vi "Get COM Descriptor from VISA.vi"(8 "error in (no error)":errorcluster, 10 "Generate error if no COM port found? (False)":bool, 11 "VISA resource name":refnum<visa-resource-name>) -> (0 "error out":errorcluster, 1 "COM port Descriptor":string, 2 "COM port":T1, 3 "VISA out":refnum<visa-resource-name>)   [LabVIEW 2020, in "Get COM Descriptor.lvlib"]
doc: "Get COM port descriptor string from VISA resource."
uses:
  Get COM Descriptor.lvlib
  COM port.ctl
  <vilib>/regexp/Match Regular Expression.xnode
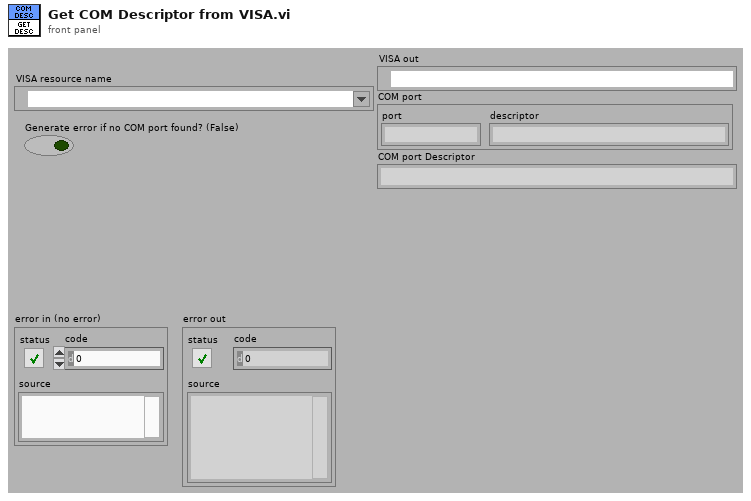
[diagram p1: front panel]
types:
  T1 = typedef "Get COM Descriptor.lvlib/COM port.ctl" = cluster{"port":string, "descriptor":string}
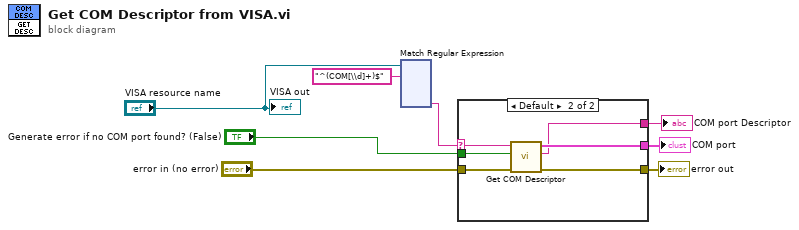
[diagram p0: block diagram]
diagram:
  n1 = xnode "Match Regular Expression"("input string"="VISA resource name", "regular expression"="^(COM[\\d]+)$") -> ("submatch 1"=w3:string)  [unwired: 4 in, 5 out]
  n2 = case shown="Default" w3 {
    selector: w3 -> [_ w12]
    tunnel: "error in (no error)" -> [w9 w15]
    tunnel: [w9 w14] -> w5
    tunnel: "Generate error if no COM port found? (False)" -> [_ w13]
    tunnel: [_ w11] -> w2
    tunnel: [_ w10] -> w1
    frame "" {
    }
    frame Default {
      n3 = call "Get COM Descriptor.vi"("error in (no error)"=w15, "Generate error if no COM port found? (False)"=w13, "COM name"=w12) -> ("error out"=w14:errorcluster, "COM port Descriptor"=w10:string, "COM port"=w11:T1)  [unwired: 6 in]
    }
  }
  "error out" <- w5
  "COM port" <- w2
  "COM port Descriptor" <- w1
  "VISA out" <- "VISA resource name"
